vi "U8 Grayscale Color.vi"() -> (4 "Color Array":u32[](array[numeric]))   [LabVIEW 2016]
doc: "Calculates the RGB Values of U8 Grayscale values."
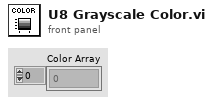
[diagram p1: front panel]
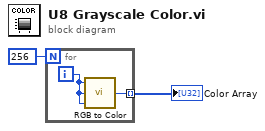
[diagram p0: block diagram]
diagram:
  n1 = for {
    N: 256 -> [_]
    tunnel: [w4] -> w1 mode=indexing
    i -> [w3]
    n2 = call <vilib>:"RGB to Color.vi"("B"=w3, "G"=w3, "R"=w3) -> ("Color"=w4:u32)
  }
  "Color Array" <- w1
